vi "Main.vi"(0 "A":dbl=5.0 format="%#_6p", 2 "Operation":T1, 5 "B":dbl=5.0 format="%#_6p", 7 "Calculate":bool, 11 "Error In":errorcluster) -> (4 "C":dbl=10.0 format="%#_6p", 15 "Error Out":errorcluster)   [LabVIEW 2019]
doc: "The VI is a simple calculator simulator that gets 2 inputs and operates based on the selection and gives one output."
uses:
  Classes/Arithemtic Operation/Arithemetic Operation.lvclass
  Typedef/Queue Operation.ctl
  Typedef/Calculator Data.ctl
  Typedef/Operations.ctl
  Typedef/Class Details.ctl
panel:
  # "Instructions:\n1. Run the VI.\n2. Specify the A and B values and select the operation to be performed.\n3. Click calculate to perform the operation.\n4. Observe the output in C indicator.\n5. Click panel close to stop the VI running."
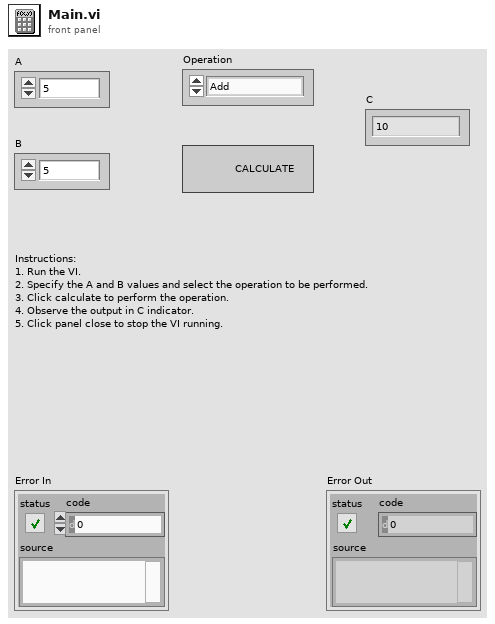
[diagram p1: front panel]
types:
  T1 = typedef "Operations.ctl" = enum16{"Add", "Subtract", "Multiply", "Divide"}
  T2 = typedef "Queue Operation.ctl" = enum16{"Create & Enqueue N", "Enqueue N", "Dequeue", "Enstack N", "Flush", "Release"}
  T3 = typedef "Calculator Data.ctl" = cluster{"A":dbl, "B":dbl, "C":dbl, "Operation":T1, "Active Class Data":refnum<class "Arithemetic Operation.lvclass">, "Class Details Array":T4[]}
  T4 = typedef "Class Details.ctl" = cluster{"Class Name":string, "Class Data":refnum<class "Arithemetic Operation.lvclass">}
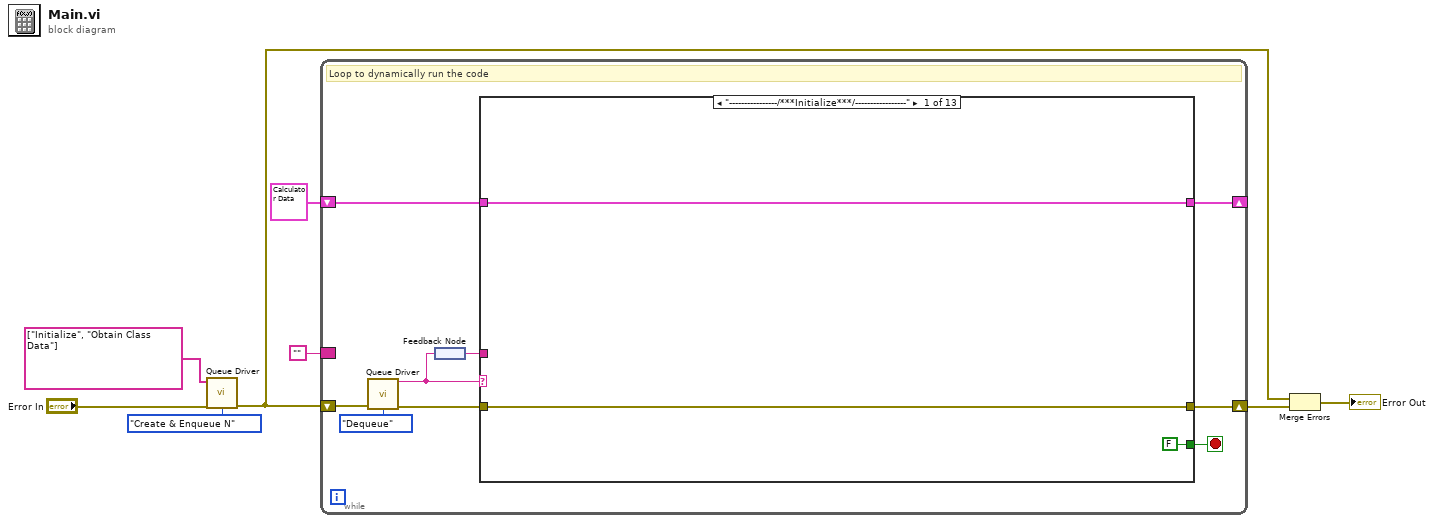
[diagram p0: block diagram]
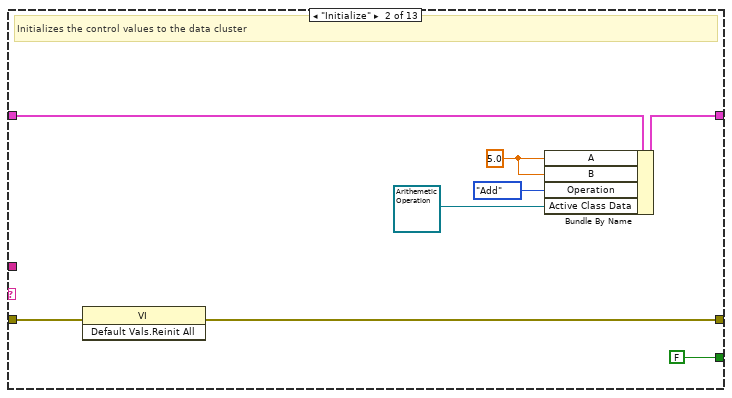
[diagram p2: hidden frame]
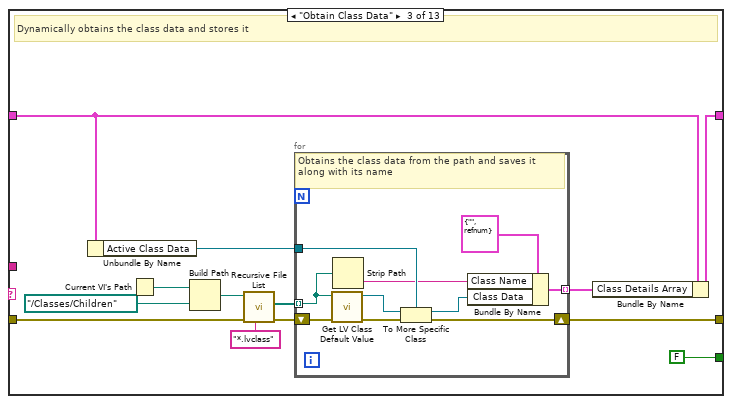
[diagram p3: hidden frame]
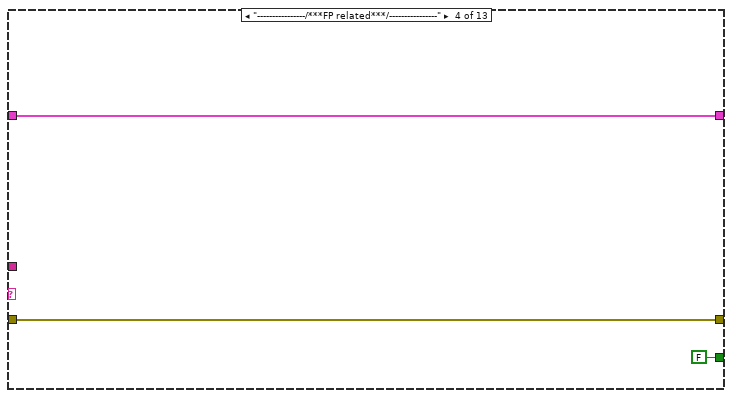
[diagram p4: hidden frame]
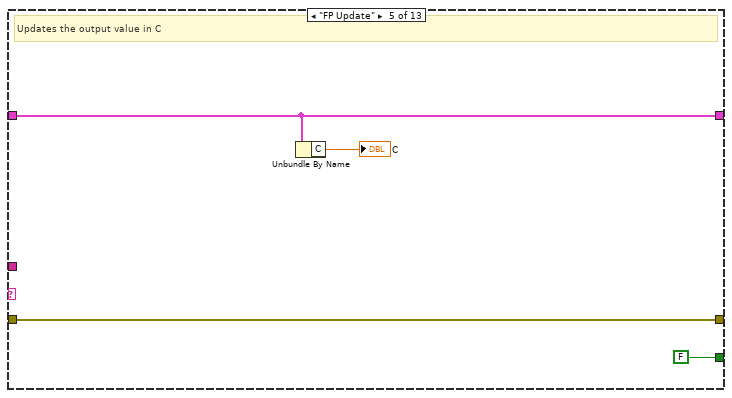
[diagram p5: hidden frame]
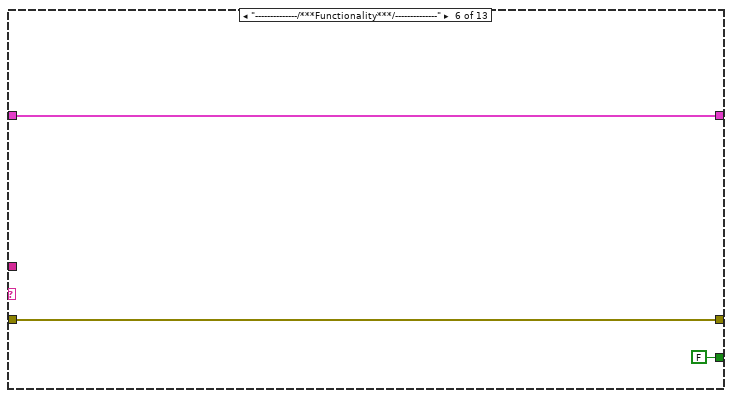
[diagram p6: hidden frame]
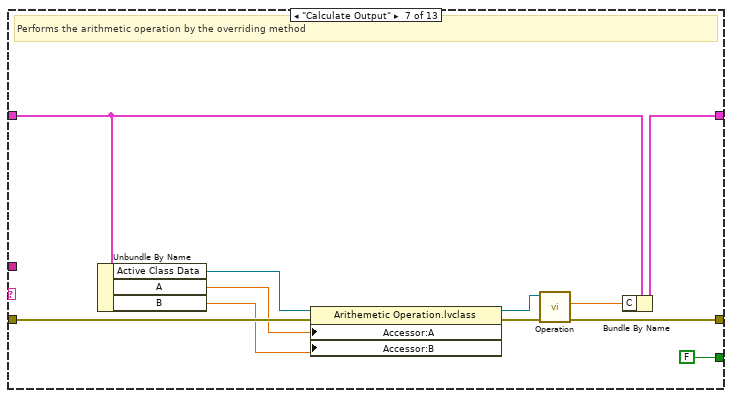
[diagram p7: hidden frame]
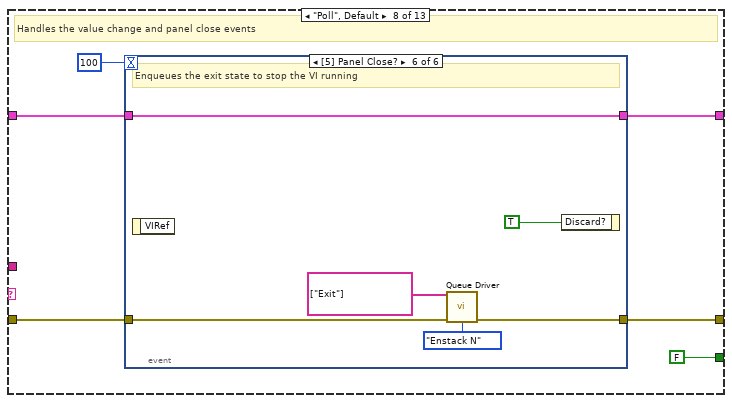
[diagram p8: hidden frame]
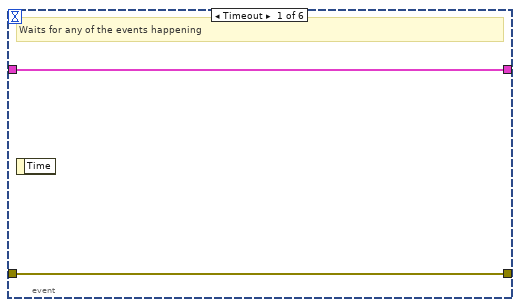
[diagram p9: hidden frame]
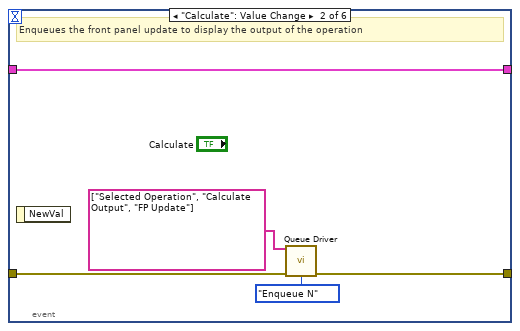
[diagram p10: hidden frame]
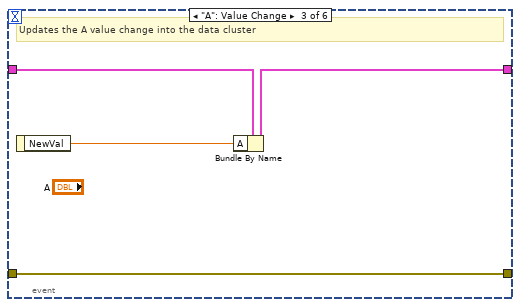
[diagram p11: hidden frame]
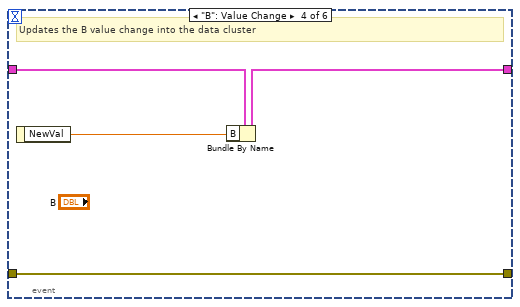
[diagram p12: hidden frame]
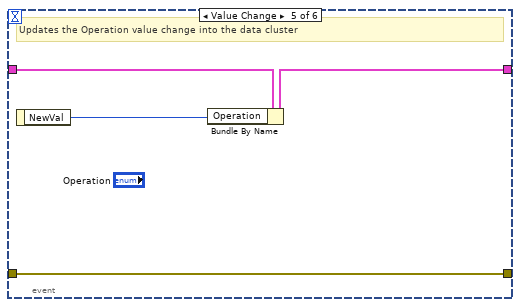
[diagram p13: hidden frame]
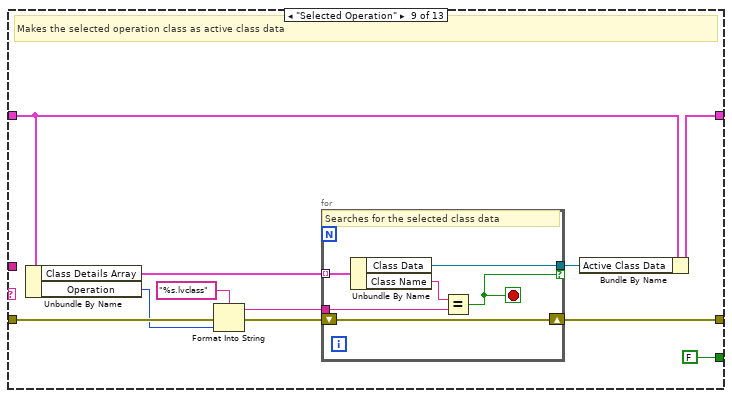
[diagram p14: hidden frame]
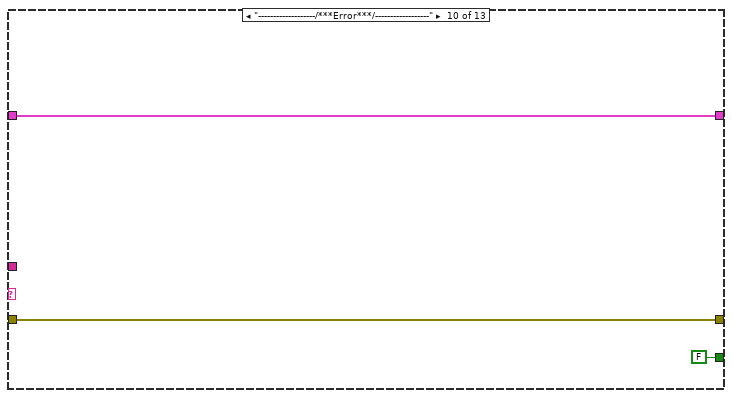
[diagram p15: hidden frame]
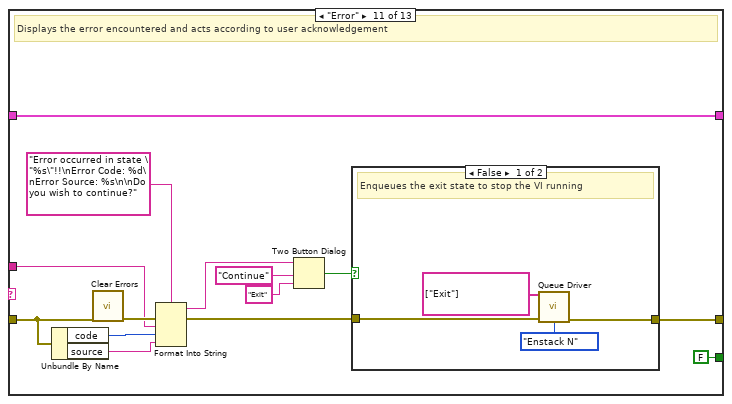
[diagram p16: hidden frame]
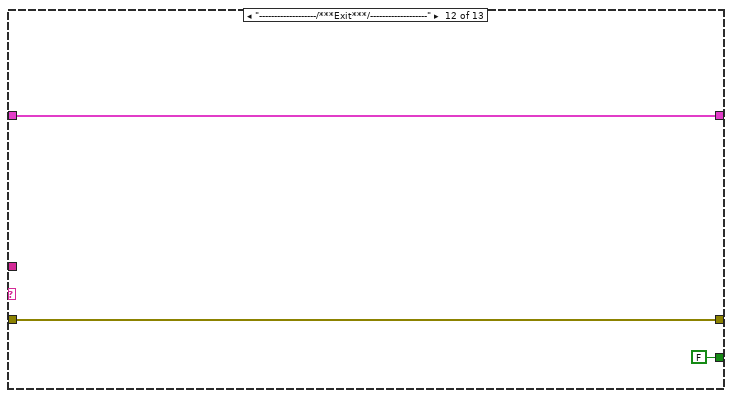
[diagram p18: hidden frame]
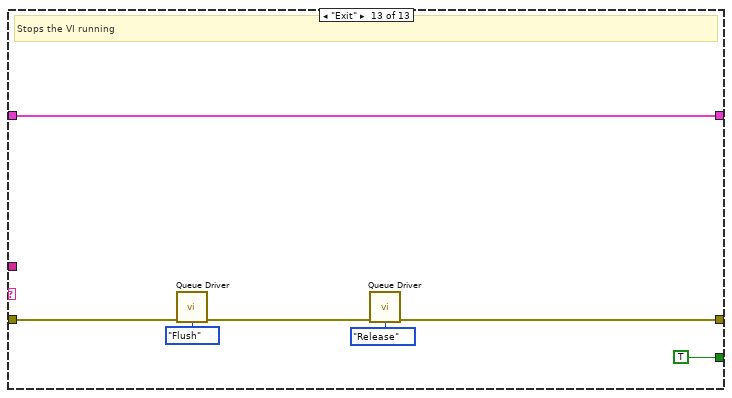
[diagram p19: hidden frame]
diagram:
  n1 = call "Queue Driver.vi"("States[]"=string[] ["Initialize", "Obtain Class Data"] ("Array of States"), "Error In"="Error In", "Operation"=Queue_Operation."Create & Enqueue N" ("Queue Operation")) -> ("Error Out"=w3:errorcluster)  [unwired: 11 in, 1 out]
  n2 = while {
    shift-right: [w13] -> _
    shift-left: T3 {"A"=0.0, "B"=0.0, "C"=0.0, "Operation"=enum."Add", "Active Class Data"=refnum, "Class Details Array"=[]} ("Calculator Data") -> [w14]
    border: "" ("Dequeue Element") -> [_]
    shift-right: [w15] -> w7
    shift-left: w3 -> [w17]
    stop <- w12 stop-if-true
    # "Loop to dynamically run the code"
    n3 = call "Queue Driver.vi"("Error In"=w17, "Operation"=Queue_Operation."Dequeue" ("Queue Operation")) -> ("Dequeue Element"=w10:string, "Error Out"=w16:errorcluster)  [unwired: 12 in]
    n4 = feedback-in #1(w10) -> ()
    n5 = feedback #1() -> (w11:string)
    n6 = case shown="\"----------------/***Initialize***/-----------------\"" w10 {
      tunnel: w16 -> [w20 w28 w41 w54 w58 w61 w72 w78 w113 w123 w129 w145 w149]
      tunnel: [w20 w24 w34 w54 w58 w61 w65 w77 w108 w123 w131 w145 w150] -> w15
      tunnel: w14 -> [w19 w27 w32 w53 w57 w60 w71 w75 w114 w122 w137 w144 w152]
      tunnel: [w19 w26 w30 w53 w57 w60 w64 w74 w111 w122 w137 w144 w152] -> w13
      tunnel: [FALSE ("Stop") FALSE ("Stop") FALSE ("Stop") FALSE ("Stop") FALSE ("Stop") FALSE ("Stop") FALSE ("Stop") FALSE ("Stop") FALSE ("Stop") FALSE ("Stop") FALSE ("Stop") FALSE ("Stop") TRUE ("Stop")] -> w12
      tunnel: w11 -> [_ _ _ _ _ _ _ _ _ _ w125 _ _]
      frame "----------------/***Initialize***/-----------------" {
      }
      frame "Initialize" {
        w23 = 5.0 ("A")
        # "Initializes the control values to the data cluster"
        n7 = invoke class="VI" method="Default Vals.Reinit All"(error in=w28) -> (error out=w24:errorcluster)  [unwired: 2 in, 2 out]
        n8 = Bundle By Name(cluster=w27, "A"=w23, "B"=w23, "Operation"=Operations."Add", "Active Class Data"=refnum<class "Arithemetic Operation.lvclass"> refnum ("Class Reference")) -> (w26:T3)
      }
      frame "Obtain Class Data" {
        # "Dynamically obtains the class data and stores it"
        n9 = Unbundle By Name(w32) -> ("Active Class Data"=w31:refnum<class "Arithemetic Operation.lvclass">)
        n10 = Current VI's Path() -> (path=w38:path)
        n11 = Build Path(base path=w38, name or relative path=path "../Classes/Children") -> (appended path=w36:path)
        n12 = call <vilib>:"Recursive File List.vi"("pattern"="*.lvclass", "error in (no error)"=w41, "Folder Path"=w36) -> ("error out"=w39:errorcluster, "All Files in Dir"=w33:path[])  [unwired: 4 in, 3 out]
        n13 = for {
          shift-right: [w49] -> w34
          shift-left: w39 -> [w51]
          tunnel: w33 -> [w46] mode=indexing
          tunnel: w31 -> [w47]
          tunnel: [w42] -> w29 mode=indexing
          # "Obtains the class data from the path and saves it along with its name"
          n14 = call <vilib>:"Get LV Class Default Value.vi"("error in (no error)"=w51, "class path"=w46) -> ("error out"=w50:errorcluster, "object"=w48:refnum<class>)  [unwired: 8 in]
          n15 = Strip Path(path=w46) -> (name=w44:string)  [unwired: 1 out]
          n16 = To More Specific Class(target class=w47, reference=w48, error in=w50) -> (specific class reference=w43:refnum<class "Arithemetic Operation.lvclass">, error out=w49:errorcluster)
          n17 = Bundle By Name(cluster=T4 {"Class Name"="", "Class Data"=refnum} ("Class Details"), "Class Name"=w44, "Class Data"=w43) -> (w42:T4)
        }
        n18 = Bundle By Name(cluster=w32, "Class Details Array"=w29) -> (w30:T3)
      }
      frame "----------------/***FP related***/----------------" {
      }
      frame "FP Update" {
        # "Updates the output value in C"
        n19 = Unbundle By Name(w57) -> ("C"=→"C":dbl)
      }
      frame "--------------/***Functionality***/--------------" {
      }
      frame "Calculate Output" {
        # "Performs the arithmetic operation by the overriding method"
        n20 = Unbundle By Name(w71) -> ("Active Class Data"=w70:refnum<class "Arithemetic Operation.lvclass">, "A"=w69:dbl, "B"=w68:dbl)
        n21 = property class="Arithemetic Operation.lvclass"(reference=w70, error in=w72, "Accessor:A"=w69, "Accessor:B"=w68) -> (reference out=w67:refnum<class "Arithemetic Operation.lvclass">, error out=w66:errorcluster)
        n22 = call-dynamic "Operation.vi"("Error In"=w66, "Arithemetic Operation in"=w67) -> ("Error Out"=w65:errorcluster, "C"=w63:dbl)  [unwired: 7 in, 1 out]
        n23 = Bundle By Name(cluster=w71, "C"=w63) -> (w64:T3)
      }
      frame "Poll", Default {
        # "Handles the value change and panel close events"
        n24 = event shown="[5] Panel Close?" {
          selector: _ -> [_ _ _ _ _ _]
          dyn-events: _ -> [_ _ _ _ _ _]
          timeout: 100 -> [_ _ _ _ _ _]
          tunnel: w78 -> [w80 w84 w86 w90 w94 w99]
          tunnel: [w80 w83 w86 w90 w94 w101] -> w77
          tunnel: w75 -> [w79 w85 w89 w93 w97 w103]
          tunnel: [w79 w85 w88 w92 w96 w103] -> w74
          event Timeout {
            # "Waits for any of the events happening"
            n25 = event-data() -> ()  [unwired: 1 in, 1 out]
          }
          event "Calculate": Value Change {
            # "Enqueues the front panel update to display the output of the operation"
            n26 = event-data() -> ()  [unwired: 1 in, 1 out]
            n27 = call "Queue Driver.vi"("States[]"=string[] ["Selected Operation", "Calculate Output", "FP Update"] ("Array of States"), "Error In"=w84, "Operation"=Queue_Operation."Enqueue N" ("Queue Operation")) -> ("Error Out"=w83:errorcluster)  [unwired: 11 in, 1 out]
          }
          event "A": Value Change {
            # "Updates the A value change into the data cluster"
            n28 = event-data() -> ("NewVal"=w87:dbl)  [unwired: 1 in]
            n29 = Bundle By Name(cluster=w89, "A"=w87) -> (w88:T3)
          }
          event "B": Value Change {
            # "Updates the B value change into the data cluster"
            n30 = event-data() -> ("NewVal"=w91:dbl)  [unwired: 1 in]
            n31 = Bundle By Name(cluster=w93, "B"=w91) -> (w92:T3)
          }
          event Value Change {
            # "Updates the Operation value change into the data cluster"
            n32 = event-data() -> ("NewVal"=w95:T1)  [unwired: 1 in]
            n33 = Bundle By Name(cluster=w97, "Operation"=w95) -> (w96:T3)
          }
          event Panel Close? {
            # "Enqueues the exit state to stop the VI running"
            n34 = event-data() -> ()  [unwired: 1 in, 1 out]
            n35 = call "Queue Driver.vi"("States[]"=string[] ["Exit"] ("Array of States"), "Error In"=w99, "Operation"=Queue_Operation."Enstack N" ("Queue Operation")) -> ("Error Out"=w101:errorcluster)  [unwired: 11 in, 1 out]
            n36 = event-data("Discard?"=TRUE) -> ()  [unwired: 1 in, 1 out]
          }
        }
      }
      frame "Selected Operation" {
        # "Makes the selected operation class as active class data"
        n37 = Unbundle By Name(w114) -> ("Class Details Array"=w107:T4[], "Operation"=w109:T1)
        n38 = Format Into String(format string="%s.lvclass", error in=w113, w109) -> (resulting string=w104:string, error out=w110:errorcluster)  [unwired: 1 in]
        n39 = for {
          shift-right: [w120] -> w108
          shift-left: w110 -> [w120]
          tunnel: w107 -> [w119] mode=indexing
          tunnel: [w118] -> w106 if=w115
          tunnel: w104 -> [w116]
          stop <- w115 stop-if-true
          # "Searches for the selected class data"
          n40 = Unbundle By Name(w119) -> ("Class Data"=w118:refnum<class "Arithemetic Operation.lvclass">, "Class Name"=w117:string)
          n41 = Equal?(x=w117, y=w116) -> (x = y?=w115:bool)
        }
        n42 = Bundle By Name(cluster=w114, "Active Class Data"=w106) -> (w111:T3)
      }
      frame "-------------------/***Error***/------------------" {
      }
      frame "Error" {
        # "Displays the error encountered and acts according to user acknowledgement"
        n43 = Unbundle By Name(w129) -> ("code"=w128:i32, "source"=w127:string)
        n44 = call <vilib>:"Clear Errors.vi"("error in (no error)"=w129) -> ("error out"=w134:errorcluster)  [unwired: 5 in, 1 out]
        n45 = Format Into String(format string="Error occurred in state \"%s\"!!\nError Code: %d\nError Source: %s\n\nDo you wish to continue?", error in=w134, w125, w128, w127) -> (resulting string=w135:string, error out=w130:errorcluster)  [unwired: 1 in]
        n46 = Two Button Dialog(message=w135, 1:"Exit" ("F button name (\"Cancel\")"), 2:"Continue" ("T button name (\"OK\")")) -> (T button?=w136:bool)
        n47 = case "Continue?" shown="False" w136 {
          tunnel: [w141 w142] -> w131
          tunnel: w130 -> [w139 w142]
          frame False {
            # "Enqueues the exit state to stop the VI running"
            n48 = call "Queue Driver.vi"("States[]"=string[] ["Exit"] ("Array of States"), "Error In"=w139, "Operation"=Queue_Operation."Enstack N" ("Queue Operation")) -> ("Error Out"=w141:errorcluster)  [unwired: 11 in, 1 out]
          }
          frame True {
            # "Continues the VI running"
          }
        }
      }
      frame "-------------------/***Exit***/-------------------" {
      }
      frame "Exit" {
        # "Stops the VI running"
        n49 = call "Queue Driver.vi"("Error In"=w149, "Operation"=Queue_Operation."Flush") -> ("Error Out"=w147:errorcluster)  [unwired: 12 in, 1 out]
        n50 = call "Queue Driver.vi"("Error In"=w147, "Operation"=Queue_Operation."Release" ("Queue Operation")) -> ("Error Out"=w150:errorcluster)  [unwired: 12 in, 1 out]
      }
    }
  }
  n51 = Merge Errors(w3, w7) -> (→"Error Out":errorcluster)
